vi "Begin.vi"() -> (0 "error out":errorcluster)   [LabVIEW 2013]
doc: "Called before other user functions, this VI is expected to open initial I/O refnums, load in file data, and do all program initialization. Notice that the <B>error out</B> terminal is simply used for data flow. Wiring it to other structures or subVIs ensures that this VI runs first."
uses:
  <vilib>/Rock Robotics/WPI/DriverStation/WPI_DriverStationRobotMode2.ctl
  <vilib>/Rock Robotics/WPI/Joystick/WPI_JoystickDeviceEnum.ctl
  <vilib>/Rock Robotics/SystemInterfaces/DIO/FPGA_DIORelayChannel.ctl
  <vilib>/Rock Robotics/SystemInterfaces/DIO/FPGA_DIOChannel.ctl
  <vilib>/Rock Robotics/SystemInterfaces/Typedef/FPGA_TypedefDigitalModule.ctl
  <vilib>/Rock Robotics/WPI/Solenoid/WPI_SolenoidChannel.ctl
  State Machine Enum.ctl
  Robot Global Data.vi
  <vilib>/Rock Robotics/WPI/Solenoid/WPI_SolenoidOpenSingle.vi
  <vilib>/Rock Robotics/WPI/Compressor/WPI_CompressorGetSetRefNum.vi
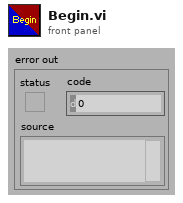
[diagram p1: front panel]
types:
  T1 = typedef "State Machine Enum.ctl" = enum16{"Init", "Actuate", "Retract"}
  T2 = typedef "WPI_SolenoidChannel.ctl" = enum8{"Solenoid 1", "Solenoid 2", "Solenoid 3", "Solenoid 4", "Solenoid 5", "Solenoid 6", "Solenoid 7", "Solenoid 8", "Invalid"}
  T3 = typedef "FPGA_TypedefDigitalModule.ctl" = enum16{"Digital Module 1", "Digital Module 2"}
  T4 = typedef "FPGA_DIOChannel.ctl" = enum8{"DIO 1", "DIO 2", "DIO 3", "DIO 4", "DIO 5", "DIO 6", "DIO 7", "DIO 8", "DIO 9", "DIO 10", "DIO 11", "DIO 12", "DIO 13", "DIO 14", "Invalid"}
  T5 = typedef "FPGA_DIORelayChannel.ctl" = enum8{"Relay 1", "Relay 2", "Relay 3", "Relay 4", "Relay 5", "Relay 6", "Relay 7", "Relay 8", "Invalid"}
  T6 = typedef "WPI_JoystickDeviceEnum.ctl" = enum16{"USB 1", "USB 2", "USB 3", "USB 4", "Kinect 1", "Kinect 2"}
  T7 = typedef "WPI_DriverStationRobotMode2.ctl" = enum16{"Autonomous Disabled", "Autonomous Enabled", "Teleop Disabled", "Teleop Enabled", "Timeout", "Finish", "Test Disabled", "Test Enabled"}
  T8 = typedef "WPI_JoystickDevRef.ctl" = cluster{"Device":T6}
  T9 = typedef "WPI_SolenoidDevRef.ctl" = cluster{"DevStatus":errorcluster, "Solenoid Module":T10, "Forward Solenoid Channel":T2, "Reverse Solenoid Channel":T2}
  T10 = typedef "FPGA_TypedefSolenoidModule.ctl" = enum16{"Solenoid Module 1", "Solenoid Module 2"}
  T11 = typedef "WPI_CompressorDevRef.ctl" = cluster{"DevStatus":errorcluster, "DigitalInputDevRef":T12, "RelayDevRef":T13}
  T12 = typedef "WPI_DigitalInputDevRef.ctl" = cluster{"DevStatus":errorcluster, "DIO Channel":T4, "Digital Module":T3}
  T13 = typedef "WPI_RelayDevRef.ctl" = cluster{"DevStatus":errorcluster, "Relay Channel":T5, "Digital Module":T3, "Relay Direction":T14}
  T14 = typedef "WPI_RelayDirection.ctl" = enum16{"Both directions", "Forward only", "Reverse only"}
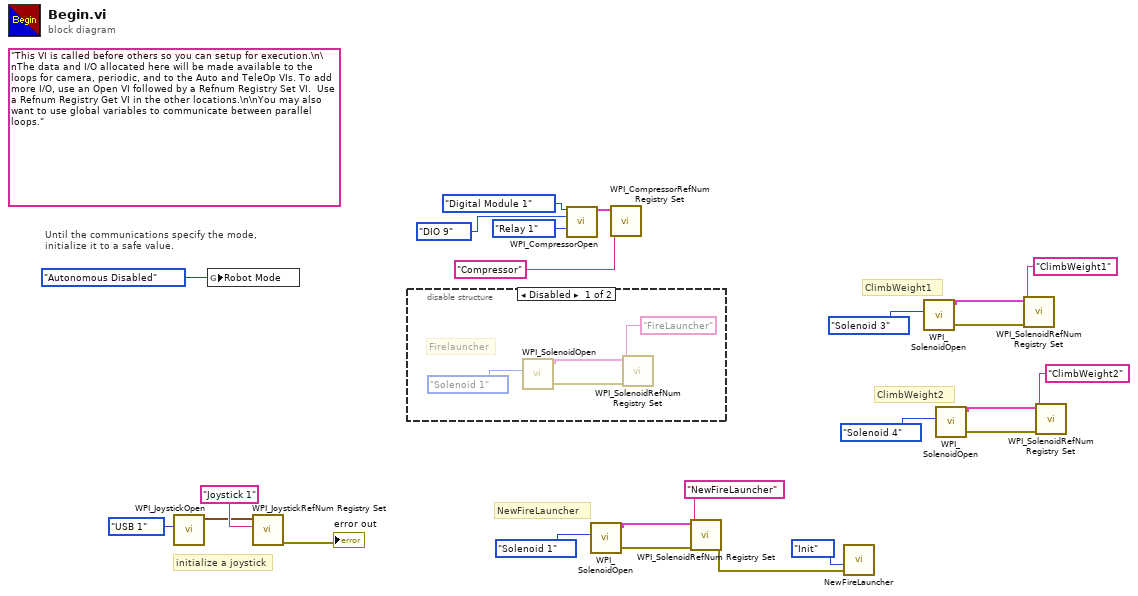
[diagram p0: block diagram]
diagram:
  (unwired) "This VI is called before others so you can setup for execution.\n\nThe data and I/O allocated here will be made available to the loops for camera, periodic, and to the Auto and TeleOp VIs. To add more I/O, use an Open VI followed by a Refnum Registry Set VI.  Use a Refnum Registry Get VI in the other locations.\n\nYou may also want to use global variables to communicate between parallel loops."
  # "NewFireLauncher"
  # "ClimbWeight2"
  # "ClimbWeight1"
  # "initialize a joystick"
  # "Until the communications specify the mode,\ninitialize it to a safe value."
  n1 = call <vilib>:"WPI_JoystickOpen.vi"("JoystickDevice"=WPI_JoystickDeviceEnum."USB 1") -> ("JoystickDevRef"=w22:T8)  [unwired: 10 in]
  n2 = global write "Robot Global Data.vi" "Robot Mode"(WPI_DriverStationRobotMode2."Autonomous Disabled" ("Robot Mode")) -> ()
  n3 = call <vilib>:"WPI_JoystickRefNum Registry Set.vi"("refnum name"="Joystick 1", "JoystickDevRef"=w22) -> ("error out"=→"error out":errorcluster)  [unwired: 8 in, 1 out]
  n4 = disable-structure shown="Disabled" {
    frame Disabled {
      # "Firelauncher"
      n5 = call-poly <vilib>:"WPI_SolenoidOpen.vi"("Solenoid Channel"=WPI_SolenoidChannel."Solenoid 1") -> ("error out"=w25:errorcluster, "SolenoidDevRef"=w27:T9)  [unwired: 9 in]
      n6 = call <vilib>:"WPI_SolenoidRefNum Registry Set.vi"("error in (no error)"=w25, "refnum name"="FireLauncher", "SolenoidDevRef"=w27) -> ()  [unwired: 7 in, 2 out]
    }
    frame Enabled {
    }
  }
  n7 = call <vilib>:"WPI_CompressorOpen.vi"("Pressure Switch Digital Module (Module 1)"=FPGA_TypedefDigitalModule."Digital Module 1" ("Pressure Switch\nand Relay Module"), "Pressure Switch DIO Channel"=FPGA_DIOChannel."DIO 9" ("Pressure Switch Channel"), "Relay Channel"=FPGA_DIORelayChannel."Relay 1") -> ("CompressorDevRef"=w16:T11)  [unwired: 2 in, 10 out]
  n8 = call-poly <vilib>:"WPI_SolenoidOpen.vi"("Solenoid Channel"=WPI_SolenoidChannel."Solenoid 1") -> ("error out"=w3:errorcluster, "SolenoidDevRef"=w5:T9)  [unwired: 9 in]
  n9 = call <vilib>:"WPI_CompressorRefNum Registry Set.vi"("refnum name"="Compressor", "CompressorDevRef"=w16) -> ()  [unwired: 8 in, 2 out]
  n10 = call <vilib>:"WPI_SolenoidRefNum Registry Set.vi"("error in (no error)"=w3, "refnum name"="NewFireLauncher", "SolenoidDevRef"=w5) -> ("error out"=w1:errorcluster)  [unwired: 7 in, 1 out]
  n11 = call "NewFireLauncher.vi"("error in (no error)"=w1, "Enum"=State_Machine_Enum."Init") -> ()  [unwired: 9 in, 1 out]
  n12 = call-poly <vilib>:"WPI_SolenoidOpen.vi"("Solenoid Channel"=WPI_SolenoidChannel."Solenoid 3") -> ("error out"=w11:errorcluster, "SolenoidDevRef"=w13:T9)  [unwired: 9 in]
  n13 = call-poly <vilib>:"WPI_SolenoidOpen.vi"("Solenoid Channel"=WPI_SolenoidChannel."Solenoid 4") -> ("error out"=w7:errorcluster, "SolenoidDevRef"=w9:T9)  [unwired: 9 in]
  n14 = call <vilib>:"WPI_SolenoidRefNum Registry Set.vi"("error in (no error)"=w11, "refnum name"="ClimbWeight1", "SolenoidDevRef"=w13) -> ()  [unwired: 7 in, 2 out]
  n15 = call <vilib>:"WPI_SolenoidRefNum Registry Set.vi"("error in (no error)"=w7, "refnum name"="ClimbWeight2", "SolenoidDevRef"=w9) -> ()  [unwired: 7 in, 2 out]
